vi "Event Nested Teardown.vi"(11 "Hello World Queue in":refnum<class "Hello World Queue.lvclass">) -> (3 "Hello World Queue out":refnum<class "Hello World Queue.lvclass">)   [LabVIEW 2021, in "Hello World Queue.lvlib" / "Hello World Queue.lvclass"]
uses:
  Hello World Queue.lvclass
  Hello World Queue.lvclass/Hello World Queue.ctl
  Actor/Queue Actor/Queue Actor.lvclass
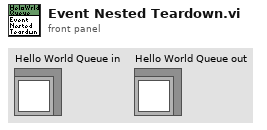
[diagram p1: front panel]
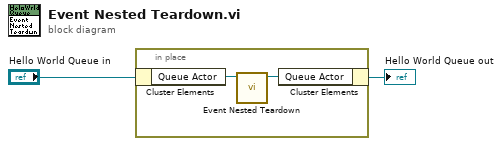
[diagram p0: block diagram]
diagram:
  n1 = in-place {
    n2 = in-place-cluster #1("Hello World Queue in") -> ("Queue Actor"=w4:refnum<class "Queue Actor.lvclass">)
    n3 = call-dynamic "Event Nested Teardown.vi"("Queue Actor in"=w4) -> ("Queue Actor out"=w3:refnum<class "Queue Actor.lvclass">)  [unwired: 10 in]
    n4 = in-place-cluster #1("Queue Actor"=w3) -> (→"Hello World Queue out":refnum<class "Hello World Queue.lvclass">)
  }
